vi "univDcimgToTif.vi"(1 "filenamesArray":path[][][](array[path])) -> (0 "conversionComplete?":bool)   [LabVIEW 2015]
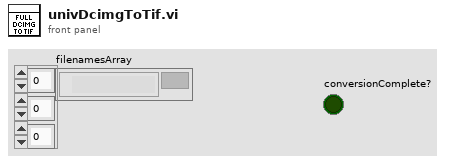
[diagram p1: front panel]
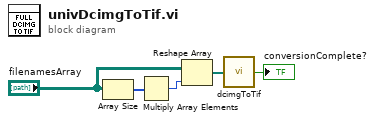
[diagram p0: block diagram]
diagram:
  n1 = Array Size(array="filenamesArray") -> (size(s)=w4:i32[])
  n2 = Multiply Array Elements(1:w4) -> (0:w3:i32)
  n3 = Reshape Array("filenamesArray", w3) -> (w5:path[])
  n4 = call "dcimgToTif.vi"("flattenedFilenamesArray"=w5) -> ("conversionComplete?"=→"conversionComplete?":bool)
